vi "CR-导丝划痕检测1 - 副本.vi"(8 "error in (no error)":errorcluster caption="错误输入（无错误）", 11 "名称或相对路径":string="Template Program") -> (0 "error in (no error) 2":errorcluster caption="错误输入（无错误）")   [LabVIEW 2017]
uses:
  Picture/SaveButtom.ctl
  <vilib>/userdefined/High Color/IMAQdx.ctl
  Global System.vi
  <vilib>/Utility/xml.llb/Write to XML File(string).vi
panel:
  in  "CCD Name":string(combo)="CCD6"
  in  "相机选择":T1="cam4" caption="Session Out CCD3"
  in  "获取图像":bool
  in  "ROI获取":bool
  in  "创建模板":bool
  in  "保存图像":bool
  out "添加的路径":path
  in  "刷新":bool
  in  "测试按钮":bool
  in  "保存按钮":bool
  in  "Main":enum32{"主参数", "模板匹配参数 ", "测试效果"}(tab)
  in  "导丝颗粒物检测1基础参数":T2={"IsNorImage"=TRUE, "Exposure Values"=100289, "ImagePath"=path "C:/Users/hedongpo/Desktop/514-hdp/Alignment Assemble System/Test Picture/B/3.bmp", "相机选择"="cam4"} caption="参数界面" {"Exposure Values" scale=0.0..200000.0}
  in  "导丝颗粒物检测1参数":T4={"Rectangle"={"Left"=0, "Top"=0, "Right"=0, "Bottom"=0, "Rotation"=0.0}, "Threshold Limits (Threshold 1)"={"Lower value"=6.0, "Upper value"=245.0}, "Keep/Remove Particles "=FALSE, "Connectivity 4/8 (8) "=TRUE, "Selection Values (Particle Filter 1)"=[{"Measurement Parameter"=35, "Range Lower Value"=80.0, "Range Upper Value"=16332.0, "Range"=FALSE, "Measurement Type"=FALSE}], "Corner Options (Feature Detection 1)"={"Detector type"=enum."Harris Corner", "Kernel size"=7, "Min Corner Point Strength"=32.0}, "Pyramid level (Feature Detection 1)"=3, "Method "=2, "Look For"=0, "Method 2"=2, "ROI Descriptor (Clamp (Rake) 1)"={"Global Rectangle"=[162, 394, 420, 1807], "Contours"=[{"ID"=enum."External", "Type"=12, "Coordinates"=[162, 394, 420, 1807, 0]}]}} {"Method" items=["clustering", "entropy", "metric", "moments", "inter-class variance"]; "Look For" items=["Bright Objects", "Dark Objects"]; "Method 2" items=["clustering", "entropy", "metric", "moments", "inter-class variance"]; "ROI Descriptor (Clamp (Rake) 1)"."Contours"."Type" items=["No Selection", "Point", "Line", "Rectangle", "Oval", "Polygon", "Freehand Region", "Annulus", "Unused2", "Unused3", "Broken Line", "Freehand Line", "Rotated Rectangle"]; "Selection Values (Particle Filter 1)"."Measurement Parameter" items=["Center of Mass X", "Center of Mass Y", "First Pixel X", "First Pixel Y", "Bounding Rect Left", "Bounding Rect Top", "Bounding Rect Right", "Bounding Rect Bottom", "Max Feret Diameter Start X", "Max Feret Diameter Start Y", "Max Feret Diameter End X", "Max Feret Diameter End Y", "Max Horiz. Segment Length Left", "Max Horiz. Segment Length Right", "Max Horiz. Segment Length Row", "-", "Bounding Rect Width", "Bounding Rect Height", "Bounding Rect Diagonal", "Perimeter", "Convex Hull Perimeter", "Holes' Perimeter", "Max Feret Diameter", "Equivalent Ellipse Major Axis", "Equivalent Ellipse Minor Axis", "Equivalent Ellipse Minor Axis (Feret)", "Equivalent Rect Long Side", "Equivalent Rect Short Side", "Equivalent Rect Diagonal", "Equivalent Rect Short Side (Feret)", "Average Horiz. Segment Length", "Average Vert. Segment Length", "Hydraulic Radius", "Waddel Disk Diameter", "-", "Area", "Holes' Area", "Particle & Holes' Area", "Convex Hull Area", "Image Area", "-", "Number of Holes", "Number of Horiz. Segments", "Number of Vert. Segments", "-", "Orientation", "Max Feret Diameter Orientation", "-", "% Area/Image Area", "% Area/(Particle & Holes' Area)", "Ratio of Equivalent Ellipse Axes", "Ratio of Equivalent Rect Sides", "-", "Elongation Factor", "Compactness Factor", "Heywood Circularity Factor", "Type Factor", "-", "Sum X", "Sum Y", "Sum XX", "Sum XY", "Sum YY", "Sum XXX", "Sum XXY", "Sum XYY", "Sum YYY", "-", "Moment of Inertia XX", "Moment of Inertia XY", "Moment of Inertia YY", "Moment of Inertia XXX", "Moment of Inertia XXY", "Moment of Inertia XYY", "Moment of Inertia YYY", "Norm. Moment of Inertia XX", "Norm. Moment of Inertia XY", "Norm. Moment of Inertia YY", "Norm. Moment of Inertia XXX", "Norm. Moment of Inertia XXY", "Norm. Moment of Inertia XYY", "Norm. Moment of Inertia YYY", "Hu Moment 1", "Hu Moment 2", "Hu Moment 3", "Hu Moment 4", "Hu Moment 5", "Hu Moment 6", "Hu Moment 7"]; "Rectangle"."Rotation" min=-90.0 max=90.0 step=1.0 format="%.2f"; "Rectangle"."Left" scale=0.0..1024.0; "Rectangle"."Right" scale=0.0..1024.0}
  out "原始图像":T5(plugin-control)
  out "颗粒物有无显示":bool
  out "Number of Features Found":i32
  in  "Feature Points Strength":string[][](table)
  in  "颗粒物个数阈值":i32
  out "路径输出":path
  in  "Vision Paramter Save Buttom":T6
  out "system time":string
  in  "取消按钮":bool
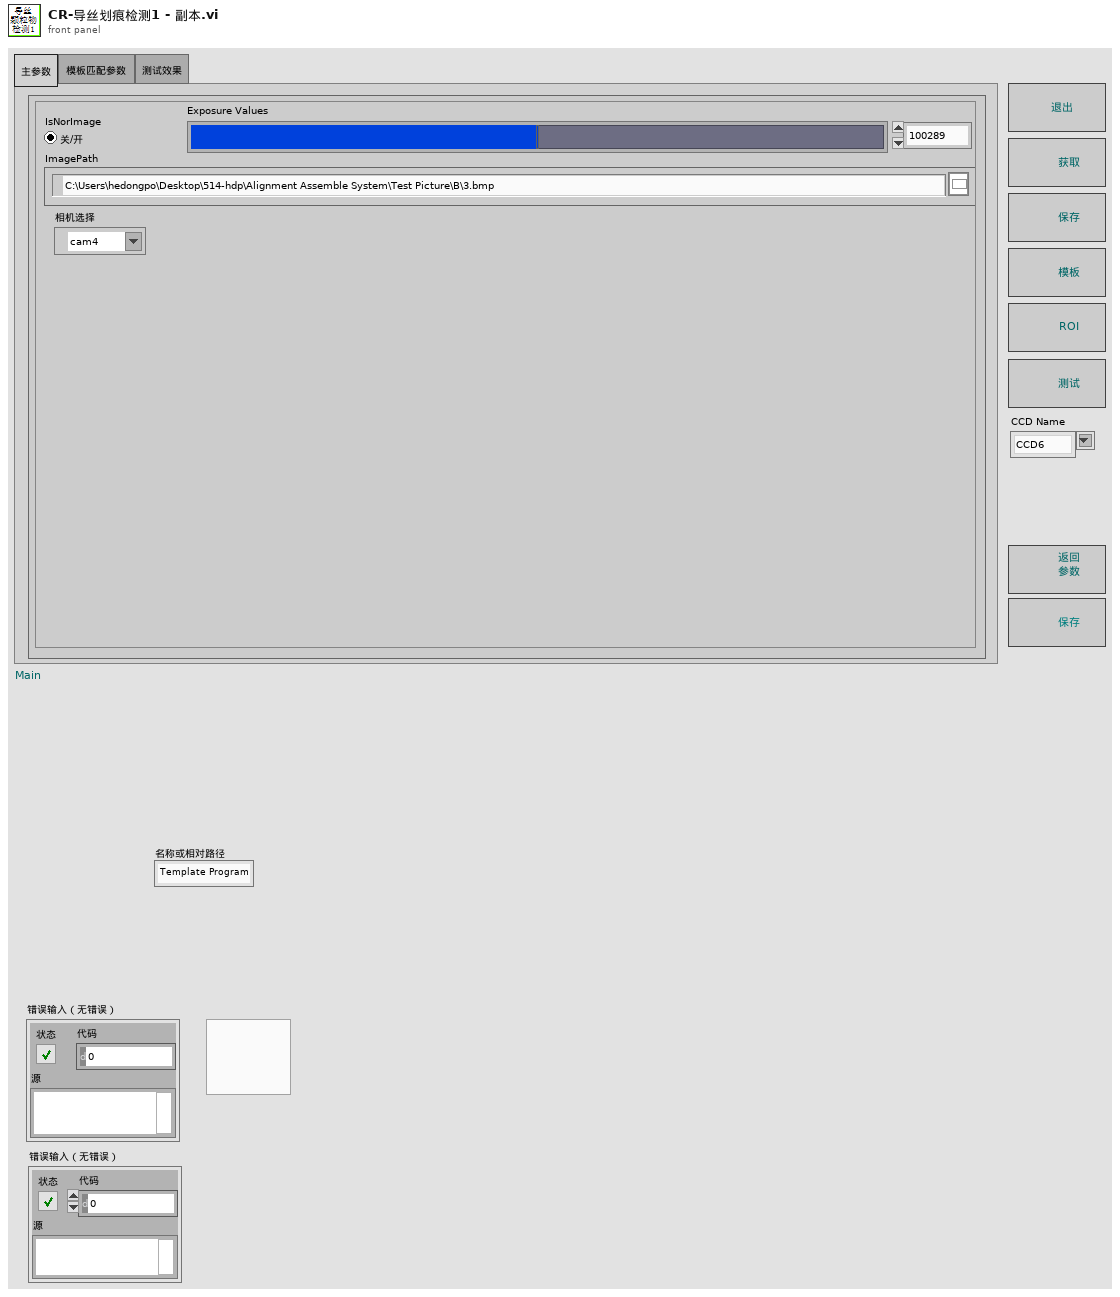
[diagram p1: front panel]
types:
  T1 = typedef "IMAQdx.ctl" = refnum<k21>
  T2 = cluster{"IsNorImage":bool, "Exposure Values":u32, "ImagePath":path, "相机选择":T1}
  T3 = typedef "IMAQ Rectangle" = cluster{"Left":i32, "Top":i32, "Right":i32, "Bottom":i32, "Rotation":dbl}
  T4 = cluster{"Rectangle":T3, "Threshold Limits (Threshold 1)":cluster{"Lower value":sgl, "Upper value":sgl}, "Keep/Remove Particles ":bool, "Connectivity 4/8 (8) ":bool, "Selection Values (Particle Filter 1)":cluster{"Measurement Parameter":i32, "Range Lower Value":dbl, "Range Upper Value":dbl, "Range":bool, "Measurement Type":bool}[], "Corner Options (Feature Detection 1)":cluster{"Detector type":enum32{"Harris Corner", "Shi-Tomasi Corner"}, "Kernel size":i32, "Min Corner Point Strength":dbl}, "Pyramid level (Feature Detection 1)":u32, "Method ":i32, "Look For":u32, "Method 2":i32, "ROI Descriptor (Clamp (Rake) 1)":cluster{"Global Rectangle":i32[], "Contours":cluster{"ID":enum32{"External", "Internal"}, "Type":u32, "Coordinates":i32[]}[]}}
  T5 = typedef "IMAQ Image.ctl" = refnum<image>
  T6 = typedef "SaveButtom.ctl" = bool
  T7 = cluster{"index":i32, "this vi":refnum<vi>, "error out":errorcluster}
  T8 = cluster{"master data":string, "priority":u16, "secondary data":string[]}
  T9 = cluster{"case name":string[], "queue array":refnum<queue>[]}
  T10 = cluster{"Global Rectangle":i32[], "Contours":cluster{"Contour Type":u32, "ROI Type":u32, "Points":i32[]}[]}
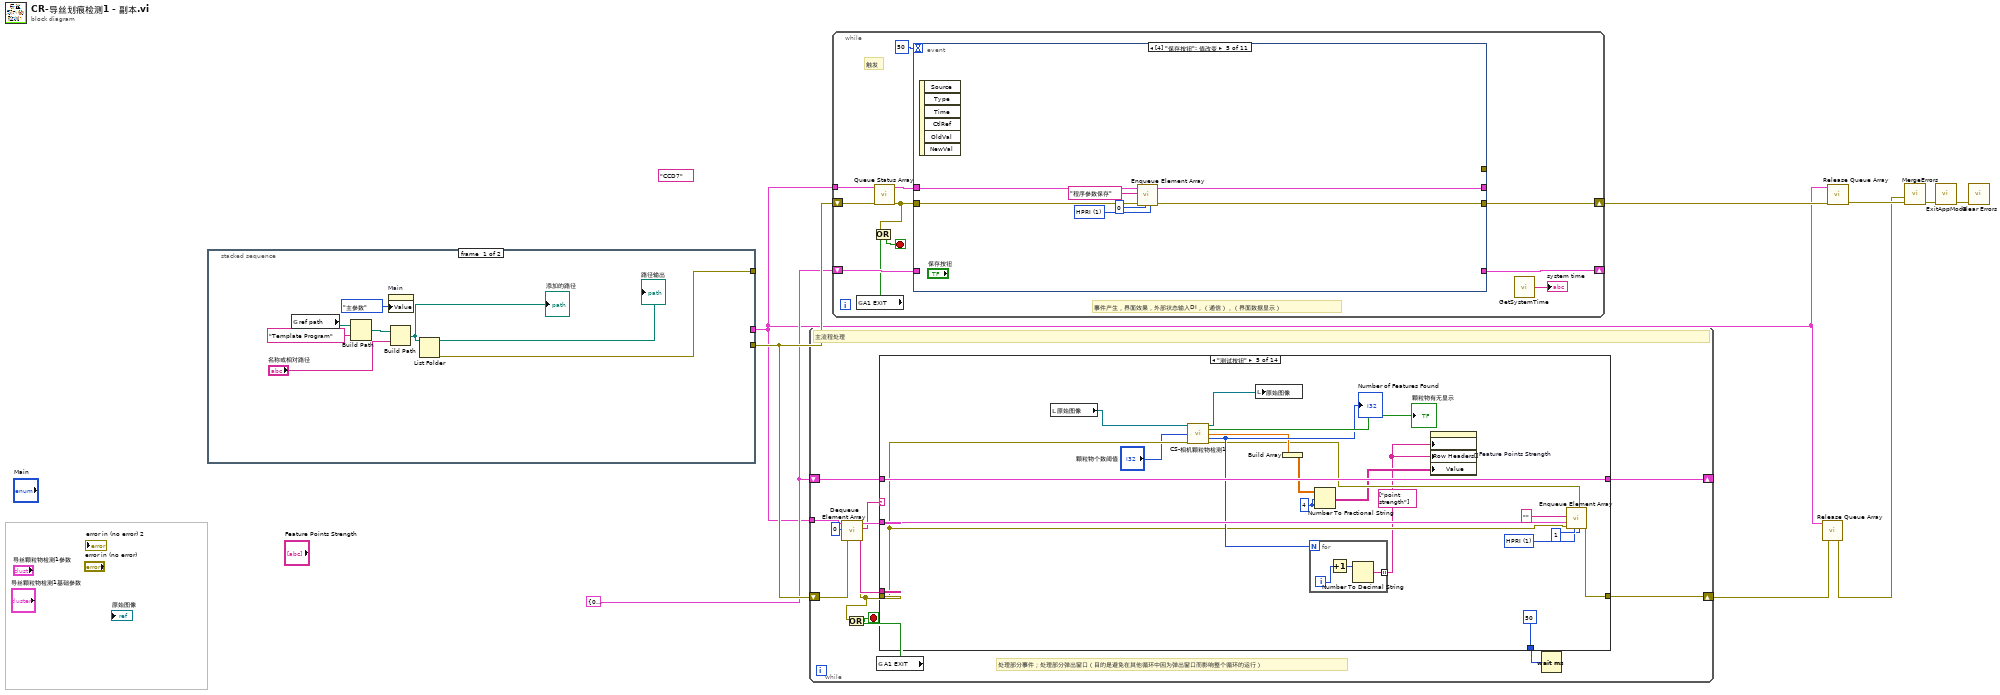
[diagram p0: block diagram]
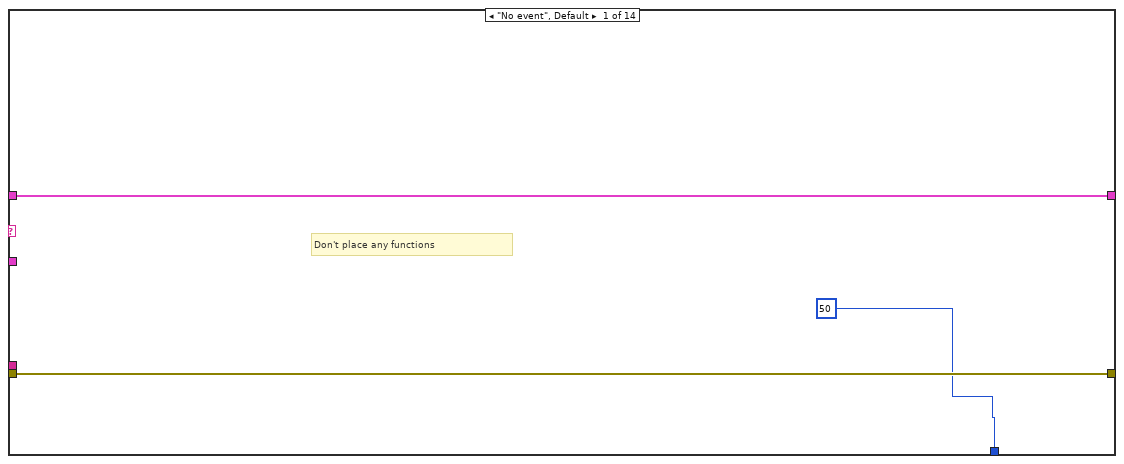
[diagram p2: hidden frame]
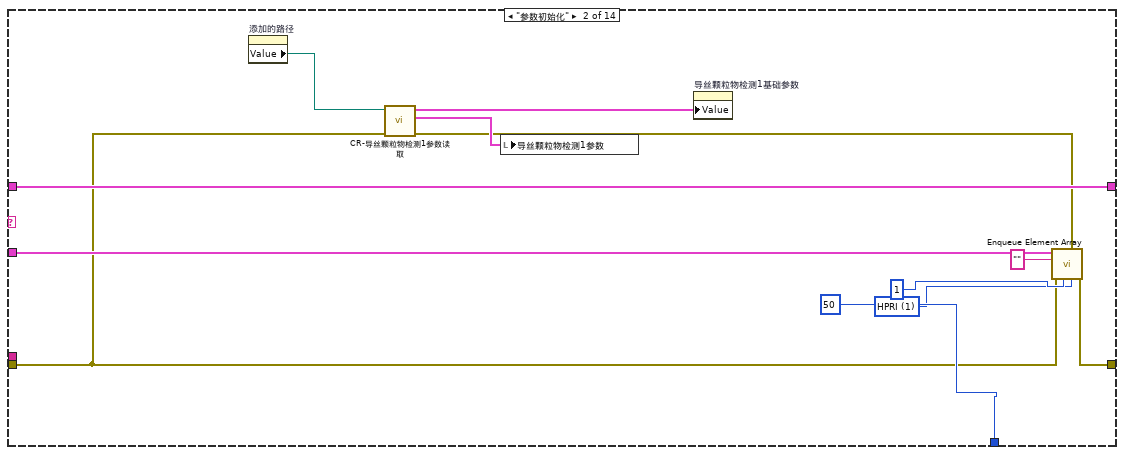
[diagram p3: hidden frame]
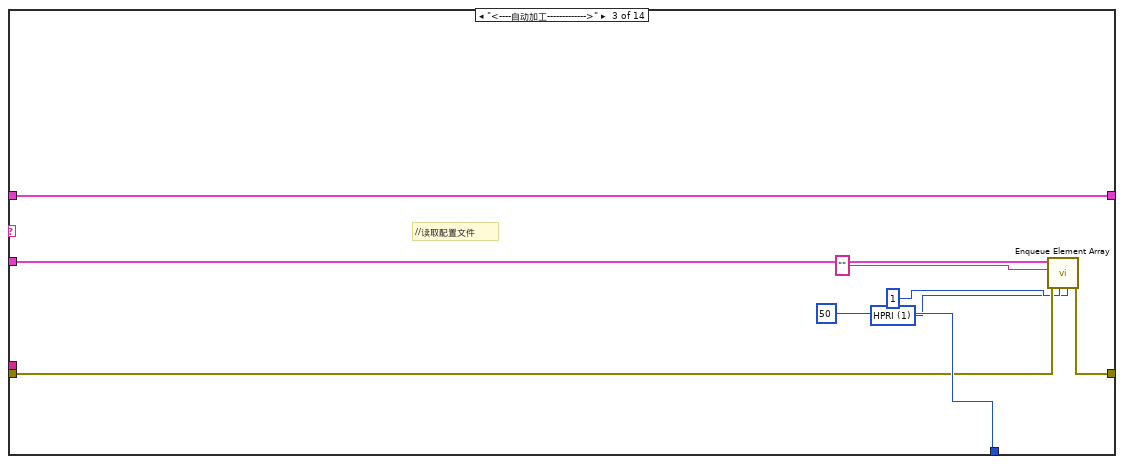
[diagram p4: hidden frame]
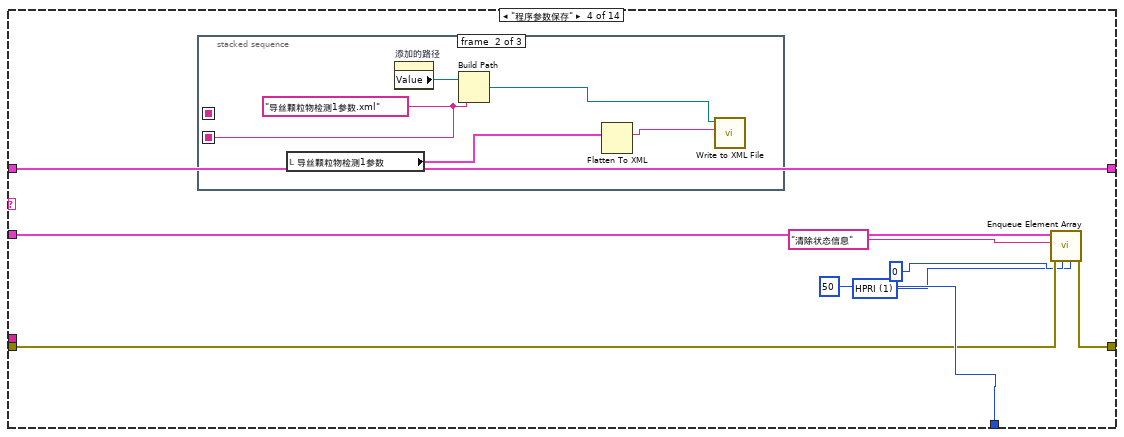
[diagram p5: hidden frame]
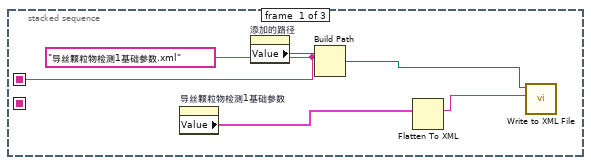
[diagram p6: hidden frame]
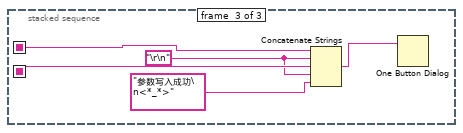
[diagram p7: hidden frame]
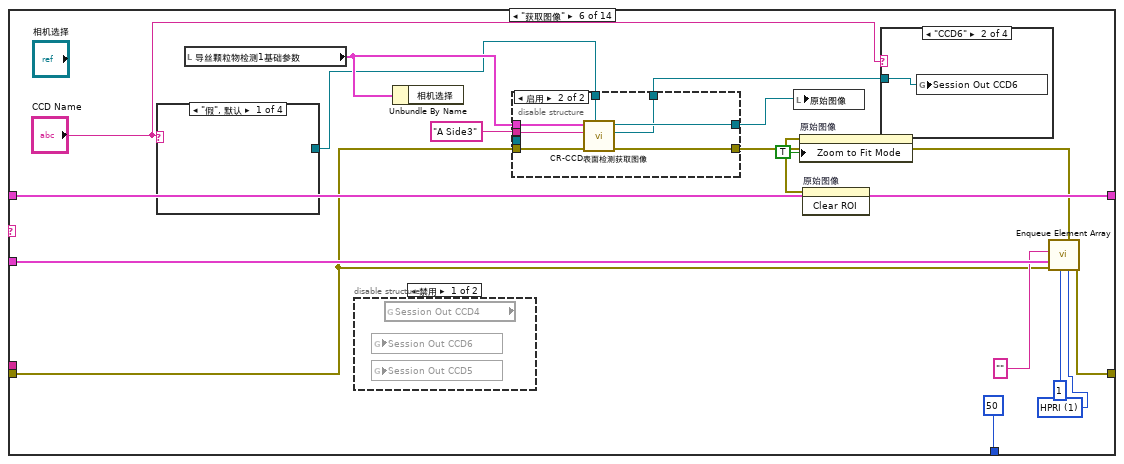
[diagram p8: hidden frame]
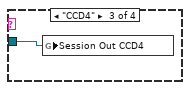
[diagram p10: hidden frame]
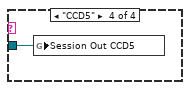
[diagram p11: hidden frame]
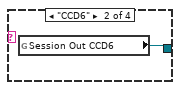
[diagram p12: hidden frame]
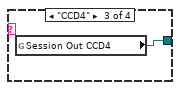
[diagram p13: hidden frame]
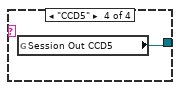
[diagram p14: hidden frame]
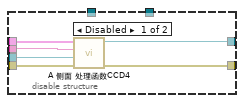
[diagram p15: hidden frame]
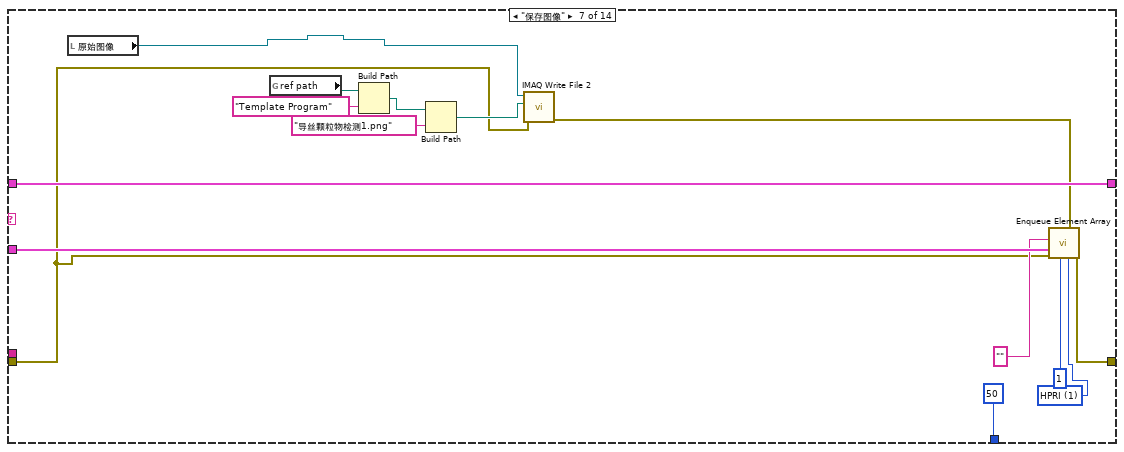
[diagram p17: hidden frame]
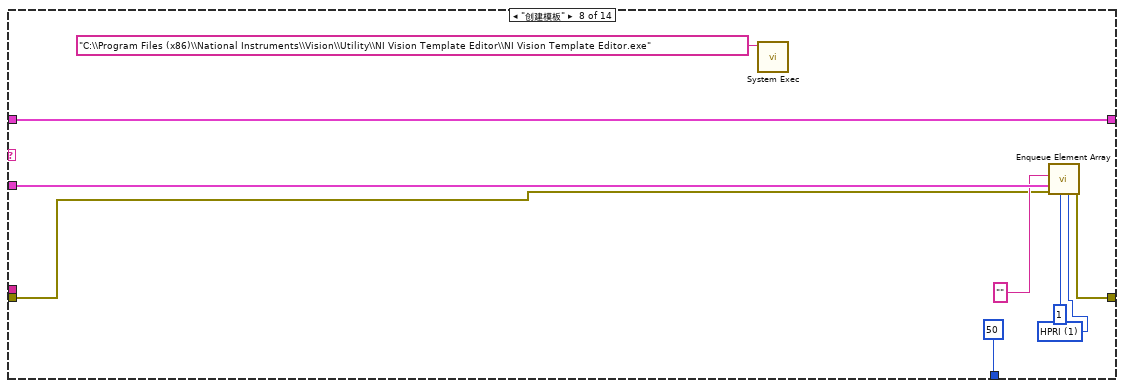
[diagram p18: hidden frame]
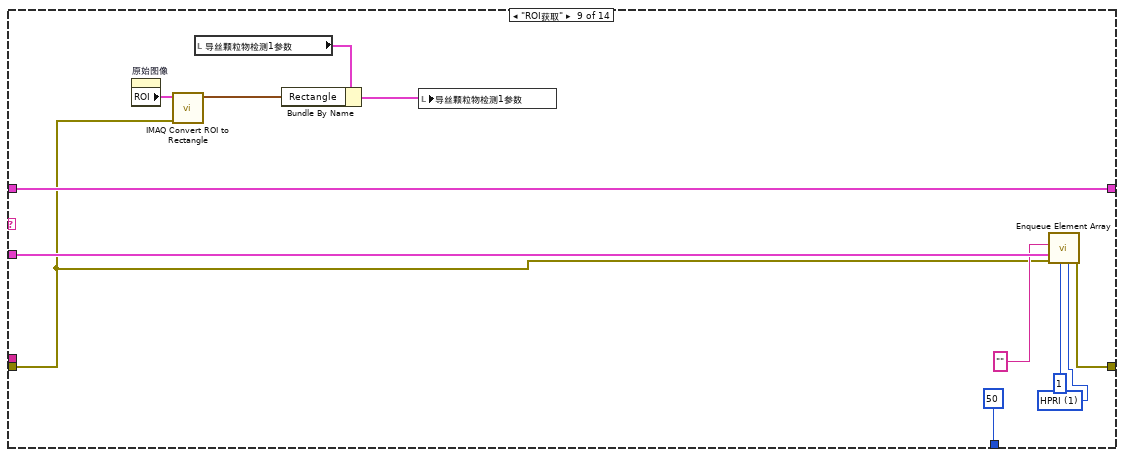
[diagram p19: hidden frame]
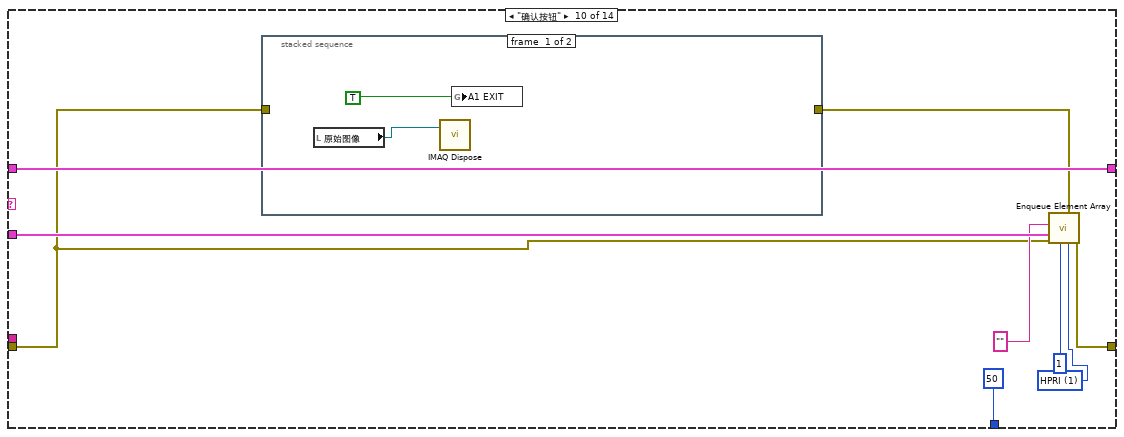
[diagram p20: hidden frame]
diagram:
  (unwired) "CCD7" ("CCD Name")
  w4 = T7 {"index"=0, "this vi"=refnum, "error out"={"status"=FALSE, "code"=0, "source"=""}} ("parameter buffer")
  n1 = stacked-sequence {
    tunnel: [w15 _] -> _
    tunnel: [_ w19] -> w5
    tunnel: [_ w18] -> w1
    frame #0 {
      n2 = global read "Global System.vi" "ref path"() -> (w13:path)
      n3 = Build Path(base path=w13, name or relative path="Template Program" ("名称或相对路径")) -> (appended path=w11:path)
      n4 = property on="Main" class="TabCtl (严格)"("Value"=enum32{"主参数", "模板匹配参数 ", "测试效果"}."主参数" ("Main")) -> ()  [unwired: 2 in, 2 out]
      n5 = Build Path(base path=w11, name or relative path="名称或相对路径") -> (appended path=w17:path)
      "添加的路径" <- w17
      n6 = List Folder(path=w17) -> (path out=→"路径输出":path, error out=w15:errorcluster)  [unwired: 3 in, 2 out]
    }
    frame #1 {
      w27 = string[] ["comm queue1", "data queue 11", "data queue 12", "data queue 13", "data queue 14"]  # queue name
      w28 = 4  # queue num
      w29 = T8 {"master data"="", "priority"=0, "secondary data"=[]}  # element data type
      n7 = call "Obtain Queue Array.vi"("queue name"=w27, "element data type"=w29, "queue num"=w28) -> ("error out"=w23:errorcluster, "queue out"=w24:T9)  [unwired: 2 in, 1 out]
      n8 = call "Enqueue Element Array.vi"("queue index"=0, "error in"=w23, "master data"="参数初始化", "queue in"=w24) -> ("error out"=w22:errorcluster, "queue out"=w21:T9)  [unwired: 6 in]
      n9 = disable-structure shown="启用" {
        disable-tunnel: w22 -> [w35 w36]
        disable-tunnel: w21 -> [w34 w37]
        disable-tunnel: "Loading Variable" ("master data") -> [w33 _]
        disable-tunnel: [w31 w36] -> w19
        disable-tunnel: [w30 w37] -> w18
        frame Disabled {
          n10 = call "Enqueue Element Array.vi"("queue index"=12, "error in"=w35, "master data"=w33, "queue in"=w34) -> ("error out"=w31:errorcluster, "queue out"=w30:T9)  [unwired: 6 in]
        }
        frame Enabled {
        }
      }
    }
  }
  n11 = while {
    shift-right: [w50] -> w3
    shift-left: w5 -> [w41]
    shift-right: [w47] -> _
    shift-left: w4 -> [w48]
    tunnel: w1 -> [w43]
    stop <- w38 stop-if-true
    # "处理部分事件；处理部分弹出窗口（目的是避免在其他循环中因为弹出窗口而影响整个循环的运行）"
    # "主流程处理"
    n12 = call "Dequeue Element Array.vi"("queue in"=w43, "queue index"=0, "error in"=w41) -> ("queue out"=w46:T9, "master data"=w45:string, "secondary data"=w44:string[], "error out"=w40:errorcluster)  [unwired: 2 in, 1 out]
    n13 = global read "Global System.vi" "A1 EXIT"() -> (w39:bool)
    n14 = Or(x=w40, y=w39) -> (x .or. y?=w38:bool)
    n15 = case shown="\"测试按钮\"" w45 {
      tunnel: w46 -> [_ w64 w72 w74 w114 w133 w167 w176 w188 w197 w210 w218 w226 w232]
      tunnel: w40 -> [w52 w54 w68 w78 w103 w125 w154 w170 w181 w191 w206 w214 w222 w229]
      tunnel: [w52 w63 w71 w80 w113 w132 w166 w175 w187 w196 w209 w217 w225 w240] -> w50
      tunnel: [50 50 50 50 50 50 50 50 50 50 50 50 50 50] -> w49
      tunnel: w48 -> [w53 w59 w69 w75 w109 w128 w162 w171 w183 w192 w207 w215 w223 w238]
      tunnel: [w53 w59 w69 w75 w109 w128 w162 w171 w183 w192 w207 w215 w223 w238] -> w47
      tunnel: w44 -> [_ _ _ _ _ _ _ _ _ _ _ _ _ _]
      frame "No event", Default {
        # "Don't place any functions"
      }
      frame "参数初始化" {
        w60 = u16 1 items=["HPRI"=1, "LPRI"=0] ("priority")
        n16 = property on="添加的路径" class="Path"() -> ("Value"=w58:path)  [unwired: 2 in, 2 out]
        n17 = call "CR-导丝颗粒物检测1参数读取.vi"("error in (no error)"=w54, "基路径"=w58) -> ("error out"=w55:errorcluster, "导丝颗粒物检测1参数"=w56:T4, "导丝颗粒物检测1基础参数"=w57:T2)  [unwired: 6 in]
        n18 = local write "导丝颗粒物检测1参数"(w56) -> ()
        n19 = property on="导丝颗粒物检测1基础参数" class="Clust (严格)"("Value"=w57) -> ()  [unwired: 2 in, 2 out]
        n20 = call "Enqueue Element Array.vi"("priority"=w60, "device error in"=w55, "queue index"=1, "error in"=w54, "master data"="" ("Element 1"), "queue in"=w64) -> ("error out"=w63:errorcluster)  [unwired: 4 in, 1 out]
      }
      frame "<----自动加工------------->" {
        w66 = u16 1 items=["HPRI"=1, "LPRI"=0] ("priority")
        # "//读取配置文件"
        n21 = call "Enqueue Element Array.vi"("priority"=w66, "queue index"=1, "error in"=w68, "master data"="" ("Element 1"), "queue in"=w72) -> ("error out"=w71:errorcluster)  [unwired: 5 in, 1 out]
      }
      frame "程序参数保存" {
        w76 = u16 1 items=["HPRI"=1, "LPRI"=0] ("priority")
        n22 = stacked-sequence {
          seq-local: [w82 _ _] -> [_ _ w95]
          seq-local: [_ w88 _] -> [_ _ w93]
          frame #0 {
            w82 = "导丝颗粒物检测1基础参数.xml" ("名称或相对路径")
            n23 = property on="导丝颗粒物检测1基础参数" class="Clust (严格)"() -> ("Value"=w85:T2)  [unwired: 2 in, 2 out]
            n24 = property on="添加的路径" class="Path"() -> ("Value"=w86:path)  [unwired: 2 in, 2 out]
            n25 = Build Path(base path=w86, name or relative path=w82) -> (appended path=w83:path)
            n26 = Flatten To XML(anything=w85) -> (xml string=w84:string)
            n27 = call-poly <vilib>:"Write to XML File.vi"("XML Input"=w84, "XML File Path"=w83) -> ()  [unwired: 7 in, 3 out]
          }
          frame #1 {
            w88 = "导丝颗粒物检测1参数.xml" ("名称或相对路径")
            n28 = local read "导丝颗粒物检测1参数"() -> (w87:T4)
            n29 = property on="添加的路径" class="Path"() -> ("Value"=w91:path)  [unwired: 2 in, 2 out]
            n30 = Build Path(base path=w91, name or relative path=w88) -> (appended path=w89:path)
            n31 = Flatten To XML(anything=w87) -> (xml string=w90:string)
            n32 = call-poly <vilib>:"Write to XML File.vi"("XML Input"=w90, "XML File Path"=w89) -> ()  [unwired: 7 in, 3 out]
          }
          frame #2 {
            w92 = "\r\n"
            n33 = Concatenate Strings(w95, w92, w93, w92, "参数写入成功\n<*_*>" ("消息")) -> (w94:string)
            n34 = One Button Dialog(message=w94) -> ()  [unwired: 1 in, 1 out]
          }
        }
        n35 = call "Enqueue Element Array.vi"("priority"=w76, "queue index"=0, "error in"=w78, "master data"="清除状态信息" ("Element 1"), "queue in"=w74) -> ("error out"=w80:errorcluster)  [unwired: 5 in, 1 out]
      }
      frame "测试按钮" {
        w105 = i16 4 ("精度(6)")
        (unwired) string[] ["point strength"] ("列首字符串[]")
        w110 = u16 1 items=["HPRI"=1, "LPRI"=0] ("priority")
        n36 = local read "原始图像"() -> (w98:T5)
        n37 = call "CS-相机颗粒物检测1.vi"("Image in"=w98, "颗粒物个数阈值"="颗粒物个数阈值", "error in (no error)"=w103) -> ("Image out"=w101:T5, "颗粒物有无显示"=→"颗粒物有无显示":bool, "颗粒物大小显示"=w106:dbl[], "Number of Features Found"=w107:i32, "error out"=w102:errorcluster)  [unwired: 6 in, 2 out]
        "Number of Features Found" <- w107
        n38 = local write "原始图像"(w101) -> ()
        n39 = Build Array(w106) -> (w104:dbl[][])
        n40 = for {
          N: w107 -> [_]
          tunnel: [w116] -> w99 mode=indexing
          i -> [w118]
          n41 = Increment(x=w118) -> (x+1=w117:i32)
          n42 = Number To Decimal String(number=w117) -> (decimal integer string=w116:string)  [unwired: 1 in]
        }
        n43 = Number To Fractional String(number=w104, width (-)=w105, precision (6)=w105) -> (F-format string=w100:string[][])  [unwired: 1 in]
        n44 = property on="Feature Points Strength" class="Tbl (严格)"("Column Headers[]"=w99, "Row Headers[]"=w99, "Value"=w100) -> ()  [unwired: 2 in, 2 out]
        n45 = call "Enqueue Element Array.vi"("priority"=w110, "device error in"=w102, "queue index"=1, "error in"=w103, "master data"="" ("Element 1"), "queue in"=w114) -> ("error out"=w113:errorcluster)  [unwired: 4 in, 1 out]
      }
      frame "获取图像" {
        w129 = u16 1 items=["HPRI"=1, "LPRI"=0] ("priority")
        n46 = case shown="\"假\", 默认" "CCD Name" {
          tunnel: [_ w138 w139 w140] -> w121
          frame "假", Default {
          }
          frame "CCD6" {
            n47 = global read "Global System.vi" "Session Out CCD6"() -> (w138:T1)
          }
          frame "CCD4" {
            n48 = global read "Global System.vi" "Session Out CCD4"() -> (w139:T1)
          }
          frame "CCD5" {
            n49 = global read "Global System.vi" "Session Out CCD5"() -> (w140:T1)
          }
        }
        n50 = local read "导丝颗粒物检测1基础参数"() -> (w122:T2)
        n51 = disable-structure shown="禁用" {
          frame Disabled {
            n52 = global read "Global System.vi" "Session Out CCD6"() -> ()  [unwired: 1 in]
            n53 = global read "Global System.vi" "Session Out CCD5"() -> ()  [unwired: 1 in]
            n54 = global read "Global System.vi" "Session Out CCD4"() -> ()  [unwired: 1 out]
          }
          frame Enabled {
          }
        }
        n55 = Unbundle By Name(w122) -> ()  [unwired: 1 out]
        n56 = disable-structure shown="启用" {
          disable-tunnel: "A Side3" ("Image Name") -> [w146 w150]
          disable-tunnel: [w145 w153] -> w126
          disable-tunnel: w125 -> [w144 w151]
          disable-tunnel: [w143 w152] -> w123
          disable-tunnel: w122 -> [w142 w149]
          disable-tunnel: _ -> [w141 _]
          disable-tunnel: w121 -> [_ w148]
          disable-tunnel: [_ w147] -> w120
          frame Disabled {
            n57 = call "A 侧面 处理函数CCD4.vi"("error in (no error)"=w144, "相机选择"=w141, "New Image"=w146, "ParamsUI"=w142) -> ("error out"=w143:errorcluster, "Image out"=w145:T5)  [unwired: 4 in, 2 out]
          }
          frame Enabled {
            n58 = call "CR-CCD表面检测获取图像.vi"("Session Out CCD2"=w148, "error in (no error)"=w151, "Image Name"=w150, "ParamsUI"=w149) -> ("error out"=w152:errorcluster, "Session Out"=w147:T1, "Image out"=w153:T5)  [unwired: 4 in, 1 out]
          }
        }
        n59 = local write "原始图像"(w126) -> ()
        n60 = property on="原始图像" class="ImageControl"(error in=w123, "Zoom to Fit Mode"=TRUE) -> ()  [unwired: 1 in, 2 out]
        n61 = invoke on="原始图像" class="ImageControl" method="Clear ROI"(error in=w123) -> ()  [unwired: 2 in, 3 out]
        n62 = case shown="\"CCD6\"" "CCD Name" {
          tunnel: w120 -> [_ w135 w136 w137]
          frame "假", Default {
          }
          frame "CCD6" {
            n63 = global write "Global System.vi" "Session Out CCD6"(w135) -> ()
          }
          frame "CCD4" {
            n64 = global write "Global System.vi" "Session Out CCD4"(w136) -> ()
          }
          frame "CCD5" {
            n65 = global write "Global System.vi" "Session Out CCD5"(w137) -> ()
          }
        }
        n66 = call "Enqueue Element Array.vi"("priority"=w129, "device error in"=w123, "queue index"=1, "error in"=w125, "master data"="" ("Element 1"), "queue in"=w133) -> ("error out"=w132:errorcluster)  [unwired: 4 in, 1 out]
      }
      frame "保存图像" {
        w163 = u16 1 items=["HPRI"=1, "LPRI"=0] ("priority")
        n67 = local read "原始图像"() -> (w155:T5)
        n68 = global read "Global System.vi" "ref path"() -> (w161:path)
        n69 = Build Path(base path=w161, name or relative path="Template Program" ("名称或相对路径")) -> (appended path=w159:path)
        n70 = Build Path(base path=w159, name or relative path="导丝颗粒物检测1.png" ("名称或相对路径")) -> (appended path=w157:path)
        n71 = call-poly "IMAQ Write File 2"("error in (no error)"=w154, "File Path"=w157, "Image"=w155) -> ("error out"=w156:errorcluster)  [unwired: 7 in, 1 out]
        n72 = call "Enqueue Element Array.vi"("priority"=w163, "device error in"=w156, "queue index"=1, "error in"=w154, "master data"="" ("Element 1"), "queue in"=w167) -> ("error out"=w166:errorcluster)  [unwired: 4 in, 1 out]
      }
      frame "创建模板" {
        w172 = u16 1 items=["HPRI"=1, "LPRI"=0] ("priority")
        n73 = call <vilib>:"System Exec.vi"("command line"="C:\\Program Files (x86)\\National Instruments\\Vision\\Utility\\NI Vision Template Editor\\NI Vision Template Editor.exe") -> ()  [unwired: 7 in, 4 out]
        n74 = call "Enqueue Element Array.vi"("priority"=w172, "queue index"=1, "error in"=w170, "master data"="" ("Element 1"), "queue in"=w176) -> ("error out"=w175:errorcluster)  [unwired: 5 in, 1 out]
      }
      frame "ROI获取" {
        w184 = u16 1 items=["HPRI"=1, "LPRI"=0] ("priority")
        n75 = property on="原始图像" class="ImageControl"() -> ("ROI"=w182:T10)  [unwired: 2 in, 2 out]
        n76 = call "IMAQ Convert ROI to Rectangle"("error in (no error)"=w181, "ROI Descriptor"=w182) -> ("Rectangle"=w179:T3)  [unwired: 7 in, 1 out]
        n77 = local read "导丝颗粒物检测1参数"() -> (w180:T4)
        n78 = Bundle By Name(cluster=w180, "Rectangle"=w179) -> (w178:T4)
        n79 = local write "导丝颗粒物检测1参数"(w178) -> ()
        n80 = call "Enqueue Element Array.vi"("priority"=w184, "queue index"=1, "error in"=w181, "master data"="" ("Element 1"), "queue in"=w188) -> ("error out"=w187:errorcluster)  [unwired: 5 in, 1 out]
      }
      frame "确认按钮" {
        w193 = u16 1 items=["HPRI"=1, "LPRI"=0] ("priority")
        n81 = stacked-sequence {
          tunnel: w191 -> [_ w202]
          tunnel: [_ w201] -> w190
          frame #0 {
            n82 = local read "原始图像"() -> (w199:T5)
            n83 = call "IMAQ Dispose"("Image"=w199) -> ()  [unwired: 5 in, 1 out]
            n84 = global write "Global System.vi" "A1 EXIT"(TRUE ("EXIT")) -> ()
          }
          frame #1 {
            n85 = control-ref of="本VI"() -> (w203:refnum<vi>)
            n86 = invoke class="VI" method="FP.Close"(reference=w203, error in=w202) -> (error out=w201:errorcluster)  [unwired: 1 in, 2 out]
          }
        }
        n87 = call "Enqueue Element Array.vi"("priority"=w193, "device error in"=w190, "queue index"=1, "error in"=w191, "master data"="" ("Element 1"), "queue in"=w197) -> ("error out"=w196:errorcluster)  [unwired: 4 in, 1 out]
      }
      frame "<-----自动加工结束--------->" {
        w204 = u16 1 items=["HPRI"=1, "LPRI"=0] ("priority")
        # "//读取配置文件"
        n88 = call "Enqueue Element Array.vi"("priority"=w204, "queue index"=1, "error in"=w206, "master data"="" ("Element 1"), "queue in"=w210) -> ("error out"=w209:errorcluster)  [unwired: 5 in, 1 out]
      }
      frame "<----------手动部分------------->" {
        w212 = u16 1 items=["HPRI"=1, "LPRI"=0] ("priority")
        # "//读取配置文件"
        n89 = call "Enqueue Element Array.vi"("priority"=w212, "queue index"=1, "error in"=w214, "master data"="" ("Element 1"), "queue in"=w218) -> ("error out"=w217:errorcluster)  [unwired: 5 in, 1 out]
      }
      frame "<--------------手动结束---------------->" {
        w220 = u16 1 items=["HPRI"=1, "LPRI"=0] ("priority")
        # "//读取配置文件"
        n90 = call "Enqueue Element Array.vi"("priority"=w220, "queue index"=1, "error in"=w222, "master data"="" ("Element 1"), "queue in"=w226) -> ("error out"=w225:errorcluster)  [unwired: 5 in, 1 out]
      }
      frame "*Emergency alarm" {
        w235 = u16 1 items=["HPRI"=1, "LPRI"=0] ("priority")
        w236 = u16 1 items=["HPRI"=1, "LPRI"=0] ("priority")
        # "发出处理急停信号的命令"
        # "发出处理急停信号的命令"
        n91 = call "Enqueue Element Array.vi"("priority"=w235, "queue index"=0, "error in"=w229, "master data"="" ("Element 1"), "queue in"=w232) -> ("error out"=w230:errorcluster, "queue out"=w231:T9)  [unwired: 5 in]
        n92 = call "SetTestInfoIndex.vi"("test info index"=13) -> ()
        n93 = call "Enqueue Element Array.vi"("priority"=w236, "queue index"=1, "error in"=w230, "master data"="" ("Element 1"), "queue in"=w231) -> ("error out"=w240:errorcluster)  [unwired: 5 in, 1 out]
      }
    }
    n94 = Wait (ms)(milliseconds to wait=w49) -> ()  [unwired: 1 out]
  }
  n95 = while {
    shift-right: [w245] -> w6
    shift-left: w5 -> [w249]
    shift-right: [w247] -> _
    shift-left: w4 -> [w248]
    tunnel: w1 -> [w251]
    stop <- w242 stop-if-true
    # "触发"
    # "事件产生，界面效果，外部状态输入DI，（通信），（界面数据显示）"
    n96 = global read "Global System.vi" "A1 EXIT"() -> (w243:bool)
    n97 = call "Queue Status Array.vi"("error in (no error)"=w249, "queue in"=w251) -> ("error out"=w244:errorcluster, "queue out"=w246:T9)  [unwired: 4 in]
    n98 = Or(x=w244, y=w243) -> (x .or. y?=w242:bool)
    n99 = event shown="[4] \"保存按钮\": 值改变" {
      selector: _ -> [_ _ _ _ _ _ _ _ _ _ _]
      dyn-events: _ -> [_ _ _ _ _ _ _ _ _ _ _]
      timeout: 50 -> [_ _ _ _ _ _ _ _ _ _ _]
      tunnel: w248 -> [w256 w264 _ _ _ _ _ _ _ _ _]
      tunnel: [w256 w264 _ _ _ _ _ _ _ _ _] -> w247
      tunnel: [errorcluster {"status"=FALSE, "code"=0, "source"=""} ("error out") _ _ _ _ _ _ _ _ _ _] -> _
      tunnel: w246 -> [w254 w263 w269 w276 w283 w291 w298 w305 w313 w321 w329]
      tunnel: w244 -> [w253 w262 w268 w275 w282 w290 w297 w304 w312 w320 w328]
      tunnel: [w253 w261 w266 w273 w280 w288 w295 w302 w310 w318 w326] -> w245
      tunnel: [w254 w260 w267 w274 w281 w289 w296 w303 w311 w319 w327] -> _
      event Timeout {
        # "不要在事件结构里面放入\"弹出窗口\"这样的VI保证该循环畅通无阻。"
        n100 = event-data() -> ()  [unwired: 1 in, 1 out]
      }
      event Panel Close? {
        w258 = u16 1 items=["HPRI"=1, "LPRI"=0] ("priority")
        n101 = event-data() -> ()  [unwired: 1 in, 4 out]
        n102 = call "Enqueue Element Array.vi"("priority"=w258, "queue index"=0, "error in"=w262, "master data"="*Exit application", "queue in"=w263) -> ("error out"=w261:errorcluster, "queue out"=w260:T9)  [unwired: 5 in]
        n103 = event-data("Discard?"=TRUE) -> ()  [unwired: 1 in, 1 out]
      }
      event Value Change {
        w271 = u16 1 items=["HPRI"=1, "LPRI"=0] ("priority")
        n104 = event-data() -> ()  [unwired: 1 in, 6 out]
        n105 = call "Enqueue Element Array.vi"("priority"=w271, "queue index"=0, "error in"=w268, "master data"="Vision Paramter Save", "queue in"=w269) -> ("error out"=w266:errorcluster, "queue out"=w267:T9)  [unwired: 5 in]
      }
      event "取消按钮": Value Change {
        w278 = u16 1 items=["HPRI"=1, "LPRI"=0] ("priority")
        n106 = event-data() -> ()  [unwired: 1 in, 6 out]
        n107 = call "Enqueue Element Array.vi"("priority"=w278, "queue index"=0, "error in"=w275, "master data"="确认按钮", "queue in"=w276) -> ("error out"=w273:errorcluster, "queue out"=w274:T9)  [unwired: 5 in]
      }
      event "保存按钮": Value Change {
        w285 = u16 1 items=["HPRI"=1, "LPRI"=0] ("priority")
        n108 = event-data() -> ()  [unwired: 1 in, 6 out]
        n109 = call "Enqueue Element Array.vi"("priority"=w285, "queue index"=0, "error in"=w282, "master data"="程序参数保存", "queue in"=w283) -> ("error out"=w280:errorcluster, "queue out"=w281:T9)  [unwired: 5 in]
      }
      event "获取图像": Value Change {
        w293 = u16 1 items=["HPRI"=1, "LPRI"=0] ("priority")
        n110 = event-data() -> ()  [unwired: 1 in, 6 out]
        n111 = property on="Main" class="TabCtl (严格)"("Value"=enum32{"主参数", "模板匹配参数 ", "测试效果"}."测试效果" ("Main")) -> ()  [unwired: 2 in, 2 out]
        n112 = call "Enqueue Element Array.vi"("priority"=w293, "queue index"=0, "error in"=w290, "master data"="获取图像", "queue in"=w291) -> ("error out"=w288:errorcluster, "queue out"=w289:T9)  [unwired: 5 in]
      }
      event "保存图像": Value Change {
        w300 = u16 1 items=["HPRI"=1, "LPRI"=0] ("priority")
        n113 = event-data() -> ()  [unwired: 1 in, 6 out]
        n114 = call "Enqueue Element Array.vi"("priority"=w300, "queue index"=0, "error in"=w297, "master data"="保存图像", "queue in"=w298) -> ("error out"=w295:errorcluster, "queue out"=w296:T9)  [unwired: 5 in]
      }
      event "创建模板": Value Change {
        w307 = u16 1 items=["HPRI"=1, "LPRI"=0] ("priority")
        n115 = event-data() -> ()  [unwired: 1 in, 6 out]
        n116 = call "Enqueue Element Array.vi"("priority"=w307, "queue index"=0, "error in"=w304, "master data"="创建模板", "queue in"=w305) -> ("error out"=w302:errorcluster, "queue out"=w303:T9)  [unwired: 5 in]
      }
      event "ROI获取": Value Change {
        w315 = u16 1 items=["HPRI"=1, "LPRI"=0] ("priority")
        n117 = event-data() -> ()  [unwired: 1 in, 6 out]
        n118 = property on="Main" class="TabCtl (严格)"("Value"=enum32{"主参数", "模板匹配参数 ", "测试效果"}."模板匹配参数 " ("Main")) -> ()  [unwired: 2 in, 2 out]
        n119 = call "Enqueue Element Array.vi"("priority"=w315, "queue index"=0, "error in"=w312, "master data"="ROI获取", "queue in"=w313) -> ("error out"=w310:errorcluster, "queue out"=w311:T9)  [unwired: 5 in]
      }
      event "测试按钮": Value Change {
        w323 = u16 1 items=["HPRI"=1, "LPRI"=0] ("priority")
        n120 = event-data() -> ()  [unwired: 1 in, 6 out]
        n121 = property on="Main" class="TabCtl (严格)"("Value"=enum32{"主参数", "模板匹配参数 ", "测试效果"}."测试效果" ("Main")) -> ()  [unwired: 2 in, 2 out]
        n122 = call "Enqueue Element Array.vi"("priority"=w323, "queue index"=0, "error in"=w320, "master data"="测试按钮", "queue in"=w321) -> ("error out"=w318:errorcluster, "queue out"=w319:T9)  [unwired: 5 in]
      }
      event "刷新": Value Change {
        n123 = event-data() -> ()  [unwired: 1 in, 6 out]
        n124 = disable-structure shown="禁用" {
          disable-tunnel: w329 -> [w333 _]
          disable-tunnel: w328 -> [w332 _]
          disable-tunnel: [w331 _] -> w327
          disable-tunnel: [w330 _] -> w326
          frame Disabled {
            w335 = u16 1 items=["HPRI"=1, "LPRI"=0] ("priority")
            # "刷新"
            n125 = call "Enqueue Element Array.vi"("priority"=w335, "queue index"=0, "error in"=w332, "master data"="刷新", "queue in"=w333) -> ("error out"=w330:errorcluster, "queue out"=w331:T9)  [unwired: 5 in]
          }
          frame Enabled {
          }
        }
        n126 = property on="Main" class="TabCtl (严格)"("Value"=enum32{"主参数", "模板匹配参数 ", "测试效果"}."模板匹配参数 " ("Main")) -> ()  [unwired: 2 in, 2 out]
      }
    }
    n127 = call "GetSystemTime.vi"() -> ("date/time string"=→"system time":string)  [unwired: 7 in]
  }
  n128 = call "Release Queue Array.vi"("error in"=w3, "queue in"=w1) -> ("error out"=w2:errorcluster)  [unwired: 2 in, 3 out]
  n129 = call "Release Queue Array.vi"("error in"=w6, "queue in"=w1) -> ("error out"=w9:errorcluster)  [unwired: 2 in, 3 out]
  n130 = call "MergeErrors.vi"("error in 3 (no error)"=w2, "error in 4 (no error)"=w9) -> ("error out"=w8:errorcluster)  [unwired: 6 in]
  n131 = call "ExitAppMode.vi"("error in (no error)"=w8) -> ("error out"=w7:errorcluster)  [unwired: 10 in]
  n132 = call <vilib>:"Clear Errors.vi"("error in (no error)"=w7) -> ()  [unwired: 5 in, 2 out]
